vi "MultiProcess.vi"(0 "VI Reference In":refnum<vi>, 2 "Label":string, 5 "Wash Array":T1[](array[typedef])=[{"Wash Option"="Underbody Wash", "Car Position"=1, "Elapsed Time"=5.0}, {"Wash Option"="Bug Remover", "Car Position"=1, "Elapsed Time"=5.0}, {"Wash Option"="Pre-Soak", "Car Position"=2, "Elapsed Time"=2.0}, {"Wash Option"="High Pressure Wash", "Car Position"=2, "Elapsed Time"=5.0}, {"Wash Option"="Low Pressure Wax", "Car Position"=2, "Elapsed Time"=5.0}, {"Wash Option"="Spot Free Rinse", "Car Position"=2, "Elapsed Time"=5.0}, {"Wash Option"="Tire Shine Foam", "Car Position"=3, "Elapsed Time"=5.0}, {"Wash Option"="Air Dry", "Car Position"=3, "Elapsed Time"=5.0}], 11 "error in":errorcluster) -> (4 "VI Reference Out":refnum<vi>, 15 "error out":errorcluster)   [LabVIEW 2016, in "CarWashTest.lvlib"]
doc: "Multi process test"
uses:
  CarWashTest.lvlib
  Controls/WashStepConfig.ctl
  APIs/Assert/AssertControlDisable/AssertDisabledAndGrayedOut.vi
  APIs/Assert/AssertControlValue/True.vi
  APIs/Stimulus/ControlValue/ValueSignalByPathString.vi
  APIs/Stimulus/ControlValue/SetValueAuto.vi
  APIs/Stimulus/ControlValue/ValueSignalLatchBooleanString.vi
  Drona.lvlib
  <vilib>/addons/_JKI Toolkits/Caraya/classes/Test/Test.lvclass
  APIs/Assert/AssertControlValue/AssertControlValue.lvlib
  APIs/Assert/AssertControlDisable/AssertControlDisable.lvlib
  APIs/Stimulus/ControlValue/ControlValue.lvlib
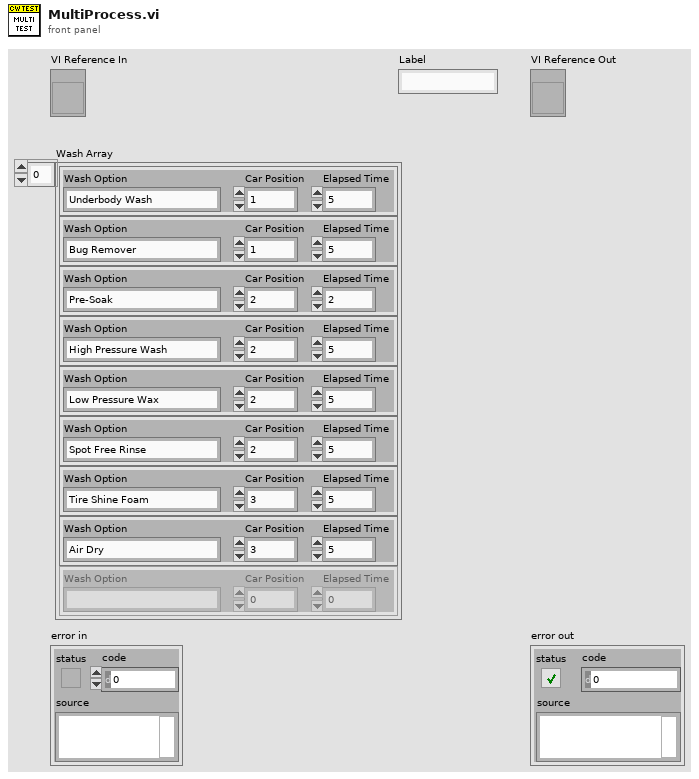
[diagram p1: front panel]
types:
  T1 = typedef "CarWashTest.lvlib/WashStepConfig.ctl" = cluster{"Wash Option":string, "Car Position":i32, "Elapsed Time":dbl}
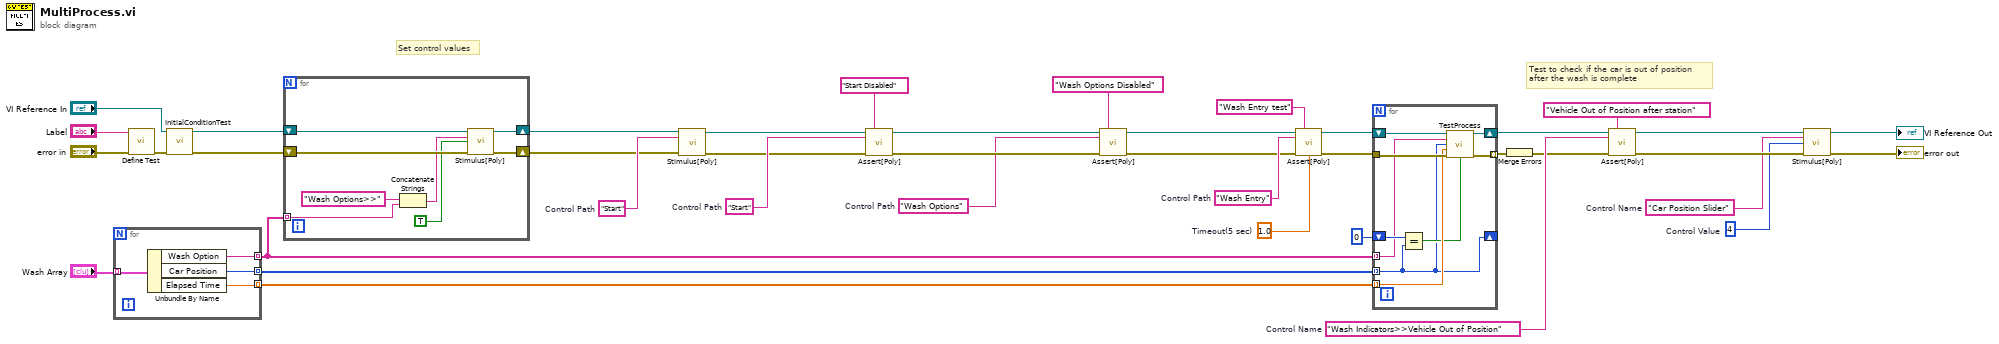
[diagram p0: block diagram]
diagram:
  w6 = "Start"  # Control Path
  w8 = "Wash Options"  # Control Path
  w33 = "Start"  # Control Path
  w26 = 4  # Control Value
  w25 = "Car Position Slider"  # Control Name
  w23 = "Wash Indicators>>Vehicle Out of Position"  # Control Name
  w22 = 1.0  # Timeout(5 sec)
  w21 = "Wash Entry"  # Control Path
  # "Set control values"
  # "Test to check if the car is out of position \nafter the wash is complete"
  n1 = for {
    tunnel: "Wash Array" -> [w44] mode=indexing
    tunnel: [w43] -> w14 mode=indexing
    tunnel: [w42] -> w16 mode=indexing
    tunnel: [w41] -> w15 mode=indexing
    n2 = Unbundle By Name(w44) -> ("Wash Option"=w43:string, "Car Position"=w42:i32, "Elapsed Time"=w41:dbl)
  }
  n3 = call <vilib>:"Define Test.vi"("error in (no error)"="error in", "Label (VI Title)"="Label") -> ("error out"=w37:errorcluster)  [unwired: 8 in, 1 out]
  n4 = call "InitialConditionTest.vi"("VI Reference In"="VI Reference In", "error in"=w37) -> ("VI Reference Out"=w40:refnum<vi>, "error out"=w38:errorcluster)  [unwired: 12 in]
  n5 = for {
    tunnel: w14 -> [w50] mode=indexing
    shift-right: [w49] -> w31
    shift-left: w40 -> [w52]
    shift-right: [w48] -> w30
    shift-left: w38 -> [w51]
    n6 = Concatenate Strings("Wash Options>>", w50) -> (w46:string)
    n7 = call-poly "Stimulus[Poly].vi"("VI Reference In"=w52, "Control Path"=w46, "Value (Signaling)"=TRUE, "error in"=w51) -> ("VI Reference Out"=w49:refnum<vi>, "error out"=w48:errorcluster)  [unwired: 10 in]
  }
  n8 = call-poly "Stimulus[Poly].vi"("VI Reference In"=w31, "Control Path"=w33, "error in"=w30) -> ("VI Reference Out"=w4:refnum<vi>, "error out"=w2:errorcluster)  [unwired: 11 in]
  n9 = call-poly "Assert[Poly].vi"("VI Reference In"=w4, "Test Label"="Start Disabled", "Control Path"=w6, "Error In"=w2) -> ("VI Reference Out"=w7:refnum<vi>, "Error Out"=w9:errorcluster)  [unwired: 9 in, 1 out]
  n10 = call-poly "Assert[Poly].vi"("VI Reference In"=w7, "Test Label"="Wash Options Disabled", "Control Path"=w8, "Error In"=w9) -> ("VI Reference Out"=w3:refnum<vi>, "Error Out"=w1:errorcluster)  [unwired: 9 in, 1 out]
  n11 = call-poly "Assert[Poly].vi"("VI Reference In"=w3, "Test Label"="Wash Entry test" ("Label"), "Control Path"=w21, "Error In"=w1, "Timeout(5 sec)"=w22) -> ("VI Reference Out"=w17:refnum<vi>, "Error Out"=w18:errorcluster)  [unwired: 8 in, 1 out]
  n12 = for {
    tunnel: w16 -> [w54] mode=indexing
    tunnel: w15 -> [w58] mode=indexing
    shift-right: [w56] -> w13
    shift-left: w17 -> [w59]
    shift-right: [w54] -> _
    shift-left: u8 0 ("Car Position") -> [w61]
    tunnel: w14 -> [w53] mode=indexing
    tunnel: w18 -> [w60]
    tunnel: [w55] -> w12 mode=indexing
    n13 = Equal?(x=w61, y=w54) -> (x = y?=w57:bool)
    n14 = call "TestProcess.vi"("VI Reference In"=w59, "Wash Option"=w53, "Car Position"=w54, "Elapsed Time"=w58, "error in"=w60, "Same Position?"=w57) -> ("VI Reference Out"=w56:refnum<vi>, "error out"=w55:errorcluster)  [unwired: 8 in]
  }
  n15 = Merge Errors(w12) -> (w20:errorcluster)
  n16 = call-poly "Assert[Poly].vi"("VI Reference In"=w13, "Test Label"="Vehicle Out of Position after station" ("Label"), "Control Path"=w23, "Error In"=w20) -> ("VI Reference Out"=w27:refnum<vi>, "Error Out"=w28:errorcluster)  [unwired: 9 in, 1 out]
  n17 = call-poly "Stimulus[Poly].vi"("VI Reference In"=w27, "Control Path"=w25, "Value (Signaling)"=w26, "error in"=w28) -> ("VI Reference Out"=→"VI Reference Out":refnum<vi>, "error out"=→"error out":errorcluster)  [unwired: 10 in]
